vi "Teleop.vi"(9 "Teleop/Auto Cluster":T1={"x Joystick"={"Device"=enum."USB 0"}, "y Joystick"={"Device"=enum."USB 1"}, "controller"={"Device"=enum."USB 2"}, "right drive encoder"={"DevStatus"={"status"=FALSE, "code"=0, "source"=""}, "EncoderIndex"=enum."Enc 0", "CounterIndex"=enum."Invalid", "DistancePerCount"=1.0, "Decoding Type"=enum."4x"}, "left drive encoder"={"DevStatus"={"status"=FALSE, "code"=0, "source"=""}, "EncoderIndex"=enum."Enc 1", "CounterIndex"=enum."Invalid", "DistancePerCount"=1.0, "Decoding Type"=enum."4x"}, "drive motors"={"DevStatus"={"status"=FALSE, "code"=0, "source"=""}, "Motors[]"=[{"DeviceStatus"={"status"=FALSE, "code"=0, "source"=""}, "Type"=enum."CAN", "PWM"={"PWM Channel"=enum."Invalid", "DeadBand"={"Name"="", "maxPositivePwm"=0, "minPositivePwm"=0, "centerPwm"=0, "maxNegativePwm"=0, "minNegativePwm"=0, "angularRange"=0}}, "CAN"={"Device Number"=1, "SetOutput VI Ref"=variant(refnum<vi> refnum), "GetOutput VI Ref"=variant(refnum<vi> refnum), "Enable VI Ref"=variant(refnum<vi> refnum), "Disable VI Ref"=variant(refnum<vi> refnum), "Data"=variant(cluster{"Ext ID":u32, "Status 0 Session Handle":u32, "Status 1 Session Handle":u32, "Param Session Handle":u32, "Param Cache ref":refnum<data-value>, "CAN Timeout":u32, "Status 2 Session Handle":u32, "Status 3 Session Handle":u32, "Inverted No WPILib":bool, "Has Configured Limit Sw":bool, "Has Configured Alt Encoder":bool, "Status 4 Session Handle":u32} {"Ext ID"=33882113, "Status 0 Session Handle"=33965, "Status 1 Session Handle"=33966, "Param Session Handle"=33969, "Param Cache ref"=refnum, "CAN Timeout"=10, "Status 2 Session Handle"=33967, "Status 3 Session Handle"=33968, "Inverted No WPILib"=TRUE, "Has Configured Limit Sw"=FALSE, "Has Configured Alt Encoder"=FALSE, "Status 4 Session Handle"=0})}, "Invert"=FALSE, "DIO PWM"={"PWM \"Enable\" Channel"=enum."Invalid", "DIOChannel"=enum."Invalid", "PWM Rate"=0.0}}, {"DeviceStatus"={"status"=FALSE, "code"=0, "source"=""}, "Type"=enum."CAN", "PWM"={"PWM Channel"=enum."Invalid", "DeadBand"={"Name"="", "maxPositivePwm"=0, "minPositivePwm"=0, "centerPwm"=0, "maxNegativePwm"=0, "minNegativePwm"=0, "angularRange"=0}}, "CAN"={"Device Number"=3, "SetOutput VI Ref"=variant(refnum<vi> refnum), "GetOutput VI Ref"=variant(refnum<vi> refnum), "Enable VI Ref"=variant(refnum<vi> refnum), "Disable VI Ref"=variant(refnum<vi> refnum), "Data"=variant(cluster{"Ext ID":u32, "Status 0 Session Handle":u32, "Status 1 Session Handle":u32, "Param Session Handle":u32, "Param Cache ref":refnum<data-value>, "CAN Timeout":u32, "Status 2 Session Handle":u32, "Status 3 Session Handle":u32, "Inverted No WPILib":bool, "Has Configured Limit Sw":bool, "Has Configured Alt Encoder":bool, "Status 4 Session Handle":u32} {"Ext ID"=33882115, "Status 0 Session Handle"=33953, "Status 1 Session Handle"=33954, "Param Session Handle"=33957, "Param Cache ref"=refnum, "CAN Timeout"=10, "Status 2 Session Handle"=33955, "Status 3 Session Handle"=33956, "Inverted No WPILib"=FALSE, "Has Configured Limit Sw"=FALSE, "Has Configured Alt Encoder"=FALSE, "Status 4 Session Handle"=0})}, "Invert"=FALSE, "DIO PWM"={"PWM \"Enable\" Channel"=enum."Invalid", "DIOChannel"=enum."Invalid", "PWM Rate"=0.0}}], "Square Inputs"=FALSE, "Max Output"=1.0}, "gyro"={"DeviceStatus"={"status"=FALSE, "code"=0, "source"=""}, "Device Number"=0, "Type"=352321536, "Device ID"=352321536, "Handle"=3028580928, "UsageFrame"=0, "Library Path"=path "libCTRE_PhoenixCCI.so"}, "drive buttons"={"Device"=enum."USB 3"}} {"gyro"."Type" items=["CAN"=352321536, "TalonSRX"=33554432]}, 10 "Match Info":T16={"Autonomous Elapsed Seconds"=0.0, "TeleOp Elapsed Seconds"=13.899, "Disabled Elapsed Seconds"=41.877, "Visited Autonomous"=FALSE, "Visited TeleOp"=TRUE, "Visited Disabled"=TRUE, "Autonomous Settings"={"Autonomous Style"=enum."Independent", "VI Refnum"=refnum}}, 11 "Call Context":T17=enum."Stop") -> ()   [LabVIEW 2019]
doc: "This VI is called for each TeleOp packet received from the DS where the robot is not disabled. It is often used to read from the joysticks and update I/O or to update setpoints for timed control loops. It should complete and return within 20 milliseconds or it may miss DS packets."
uses:
  <vilib>/Rock Robotics/WPI/DriverStation/WPI_DriverStationDerivedRobotMode.ctl
  <vilib>/Rock Robotics/WPI/DriverStation/WPI_DriverStationMatch Info.ctl
  teleop auto cluster.ctl
  <vilib>/Rock Robotics/WPI/Joystick/WPI_JoystickDevRef.ctl
  <vilib>/Rock Robotics/WPI/Joystick/WPI_JoystickDeviceEnum.ctl
  <vilib>/Rock Robotics/WPI/Encoder/WPI_EncoderDevRef.ctl
  <vilib>/Rock Robotics/SystemInterfaces/Encoder/FPGA_EncoderIdx.ctl
  <vilib>/Rock Robotics/SystemInterfaces/Counter/FPGA_CounterCtrSystemIndex.ctl
  <vilib>/Rock Robotics/WPI/Encoder/WPI_EncoderType.ctl
  <vilib>/Rock Robotics/WPI/RobotDrive/WPI_RobotDriveDevRef.ctl
  <vilib>/Rock Robotics/WPI/MotorControl/WPI_MotorControlDeviceRef.ctl
  <vilib>/Rock Robotics/WPI/MotorControl/WPI_MotorControlType.ctl
  <vilib>/Rock Robotics/SystemInterfaces/DIO/FPGA_DIOPWMChannel.ctl
  <vilib>/Rock Robotics/WPI/PWM/WPI_PWMDeadband.ctl
  <vilib>/Rock Robotics/SystemInterfaces/DIO/FPGA_DIOChannel.ctl
  <vilib>/Rock Robotics/WPI/ThirdParty/Phoenix-LabVIEW/Pigeon IMU/CTRE_PigeonIMU_DeviceRef.ctl
  <vilib>/Rock Robotics/WPI/ThirdParty/Phoenix-LabVIEW/Pigeon IMU/CTRE_PigeonIMU_ConnectionType.ctl
  GlobalVariables.vi
  <vilib>/Rock Robotics/WPI/RobotDrive/WPI_RobotDriveArcadeDrive_Standard(NoSaturation).vi
panel:
  out "Static Setpoint":bool=TRUE
  in  "Elevator Manual":dbl=0.1
  # "false is layup\ntrue is trench shot"
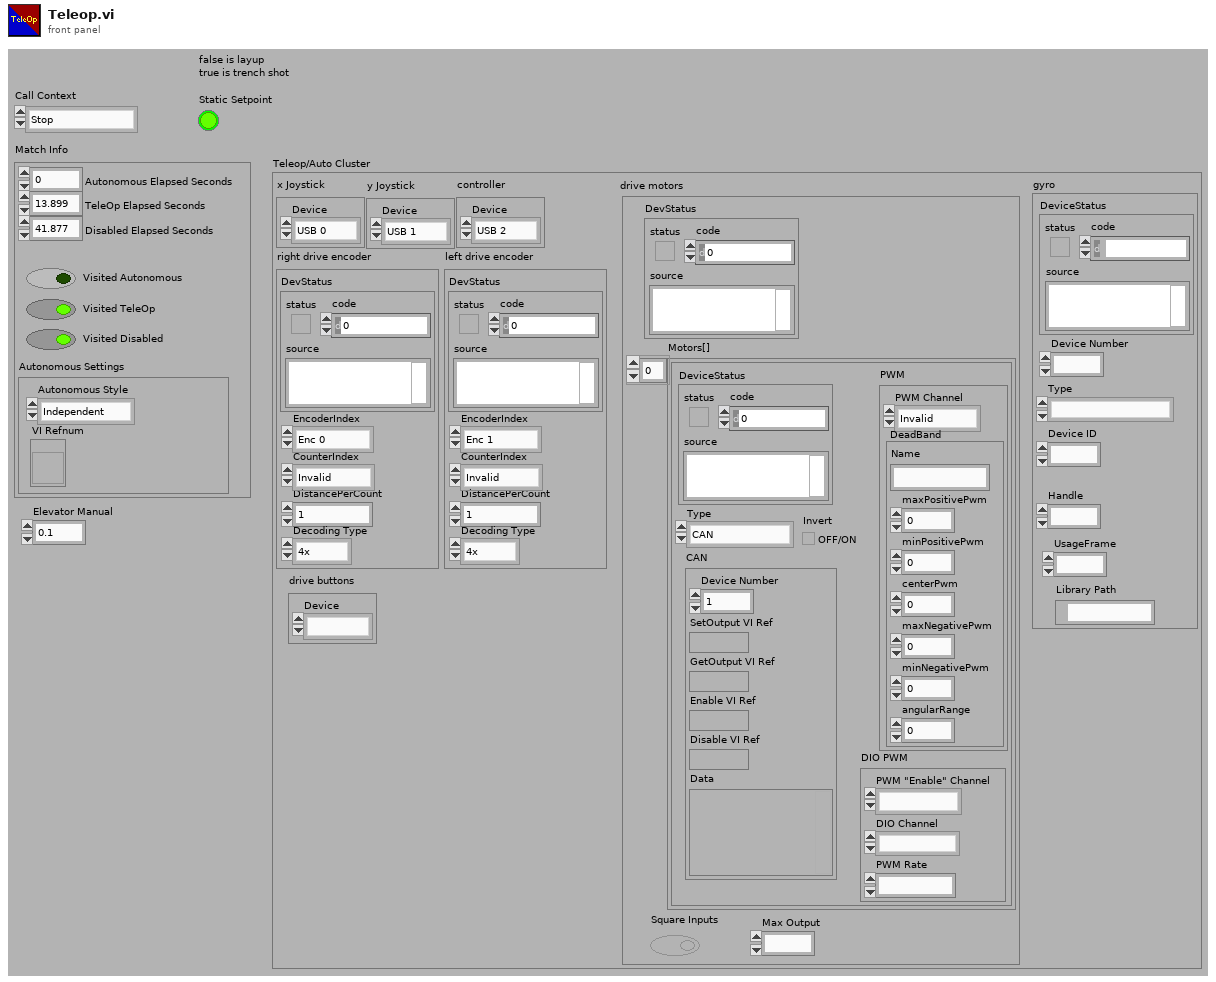
[diagram p1: front panel]
types:
  T1 = typedef "teleop auto cluster.ctl" = cluster{"x Joystick":T2, "y Joystick":T2, "controller":T2, "right drive encoder":T4, "left drive encoder":T4, "drive motors":T8, "gyro":T14, "drive buttons":T2}
  T2 = typedef "WPI_JoystickDevRef.ctl" = cluster{"Device":T3}
  T3 = typedef "WPI_JoystickDeviceEnum.ctl" = enum16{"USB 0", "USB 1", "USB 2", "USB 3", "USB 4", "USB 5"}
  T4 = typedef "WPI_EncoderDevRef.ctl" = cluster{"DevStatus":errorcluster, "EncoderIndex":T5, "CounterIndex":T6, "DistancePerCount":dbl, "Decoding Type":T7}
  T5 = typedef "FPGA_EncoderIdx.ctl" = enum8{"Enc 0", "Enc 1", "Enc 2", "Enc 3", "Enc 4", "Enc 5", "Enc 6", "Enc 7", "Invalid"}
  T6 = typedef "FPGA_CounterCtrSystemIndex.ctl" = enum8{"Ctr 0", "Ctr 1", "Ctr 2", "Ctr 3", "Ctr 4", "Ctr 5", "Ctr 6", "Ctr 7", "Invalid"}
  T7 = typedef "WPI_EncoderType.ctl" = enum16{"1x", "2x", "4x"}
  T8 = typedef "WPI_RobotDriveDevRef.ctl" = cluster{"DevStatus":errorcluster, "Motors[]":T9[], "Square Inputs":bool, "Max Output":dbl}
  T9 = typedef "WPI_MotorControlDeviceRef.ctl" = cluster{"DeviceStatus":errorcluster, "Type":T10, "PWM":cluster{"PWM Channel":T11, "DeadBand":T12}, "CAN":cluster{"Device Number":u8, "SetOutput VI Ref":variant, "GetOutput VI Ref":variant, "Enable VI Ref":variant, "Disable VI Ref":variant, "Data":variant}, "Invert":bool, "DIO PWM":cluster{"PWM \"Enable\" Channel":T11, "DIOChannel":T13, "PWM Rate":dbl}}
  T10 = typedef "WPI_MotorControlType.ctl" = enum16{"PWM", "CAN", "DIO PWM"}
  T11 = typedef "FPGA_DIOPWMChannel.ctl" = enum8{"PWM 0", "PWM 1", "PWM 2", "PWM 3", "PWM 4", "PWM 5", "PWM 6", "PWM 7", "PWM 8", "PWM 9", "PWM MXP 0", "PWM MXP 1", "PWM MXP 2", "PWM MXP 3", "PWM MXP 4", "PWM MXP 5", "PWM MXP 6", "PWM MXP 7", "PWM MXP 8", "PWM MXP 9", "Invalid"}
  T12 = typedef "WPI_PWMDeadband.ctl" = cluster{"Name":string, "maxPositivePwm":i32, "minPositivePwm":i32, "centerPwm":i32, "maxNegativePwm":i32, "minNegativePwm":i32, "angularRange":u16}
  T13 = typedef "FPGA_DIOChannel.ctl" = enum8{"DIO 0", "DIO 1", "DIO 2", "DIO 3", "DIO 4", "DIO 5", "DIO 6", "DIO 7", "DIO 8", "DIO 9", "DIO MXP 0", "DIO MXP 1", "DIO MXP 2", "DIO MXP 3", "DIO MXP 4", "DIO MXP 5", "DIO MXP 6", "DIO MXP 7", "DIO MXP 8", "DIO MXP 9", "DIO MXP 10", "DIO MXP 11", "DIO MXP 12", "DIO MXP 13", "DIO MXP 14", "DIO MXP 15", "SPI Port CS1", "SPI Port CS2", "SPI Port CS3", "SPI Port MISO", "SPI Port MOSI", "Invalid"}
  T14 = typedef "CTRE_PigeonIMU_DeviceRef.ctl" = cluster{"DeviceStatus":errorcluster, "Device Number":u8, "Type":T15, "Device ID":u32, "Handle":u64, "UsageFrame":u32, "Library Path":path}
  T15 = typedef "CTRE_PigeonIMU_ConnectionType.ctl" = u32
  T16 = typedef "WPI_DriverStationMatch Info.ctl" = cluster{"Autonomous Elapsed Seconds":dbl, "TeleOp Elapsed Seconds":dbl, "Disabled Elapsed Seconds":dbl, "Visited Autonomous":bool, "Visited TeleOp":bool, "Visited Disabled":bool, "Autonomous Settings":cluster{"Autonomous Style":enum16{"Iterative", "Independent"}, "VI Refnum":refnum<vi>}}
  T17 = typedef "WPI_DriverStationDerivedRobotMode.ctl" = enum16{"Init", "Execute", "Stop"}
  T18 = enum16{"ground protect", "ground pickup", "control panel", "shooting", "climb", "unjam", "intake shoot"}
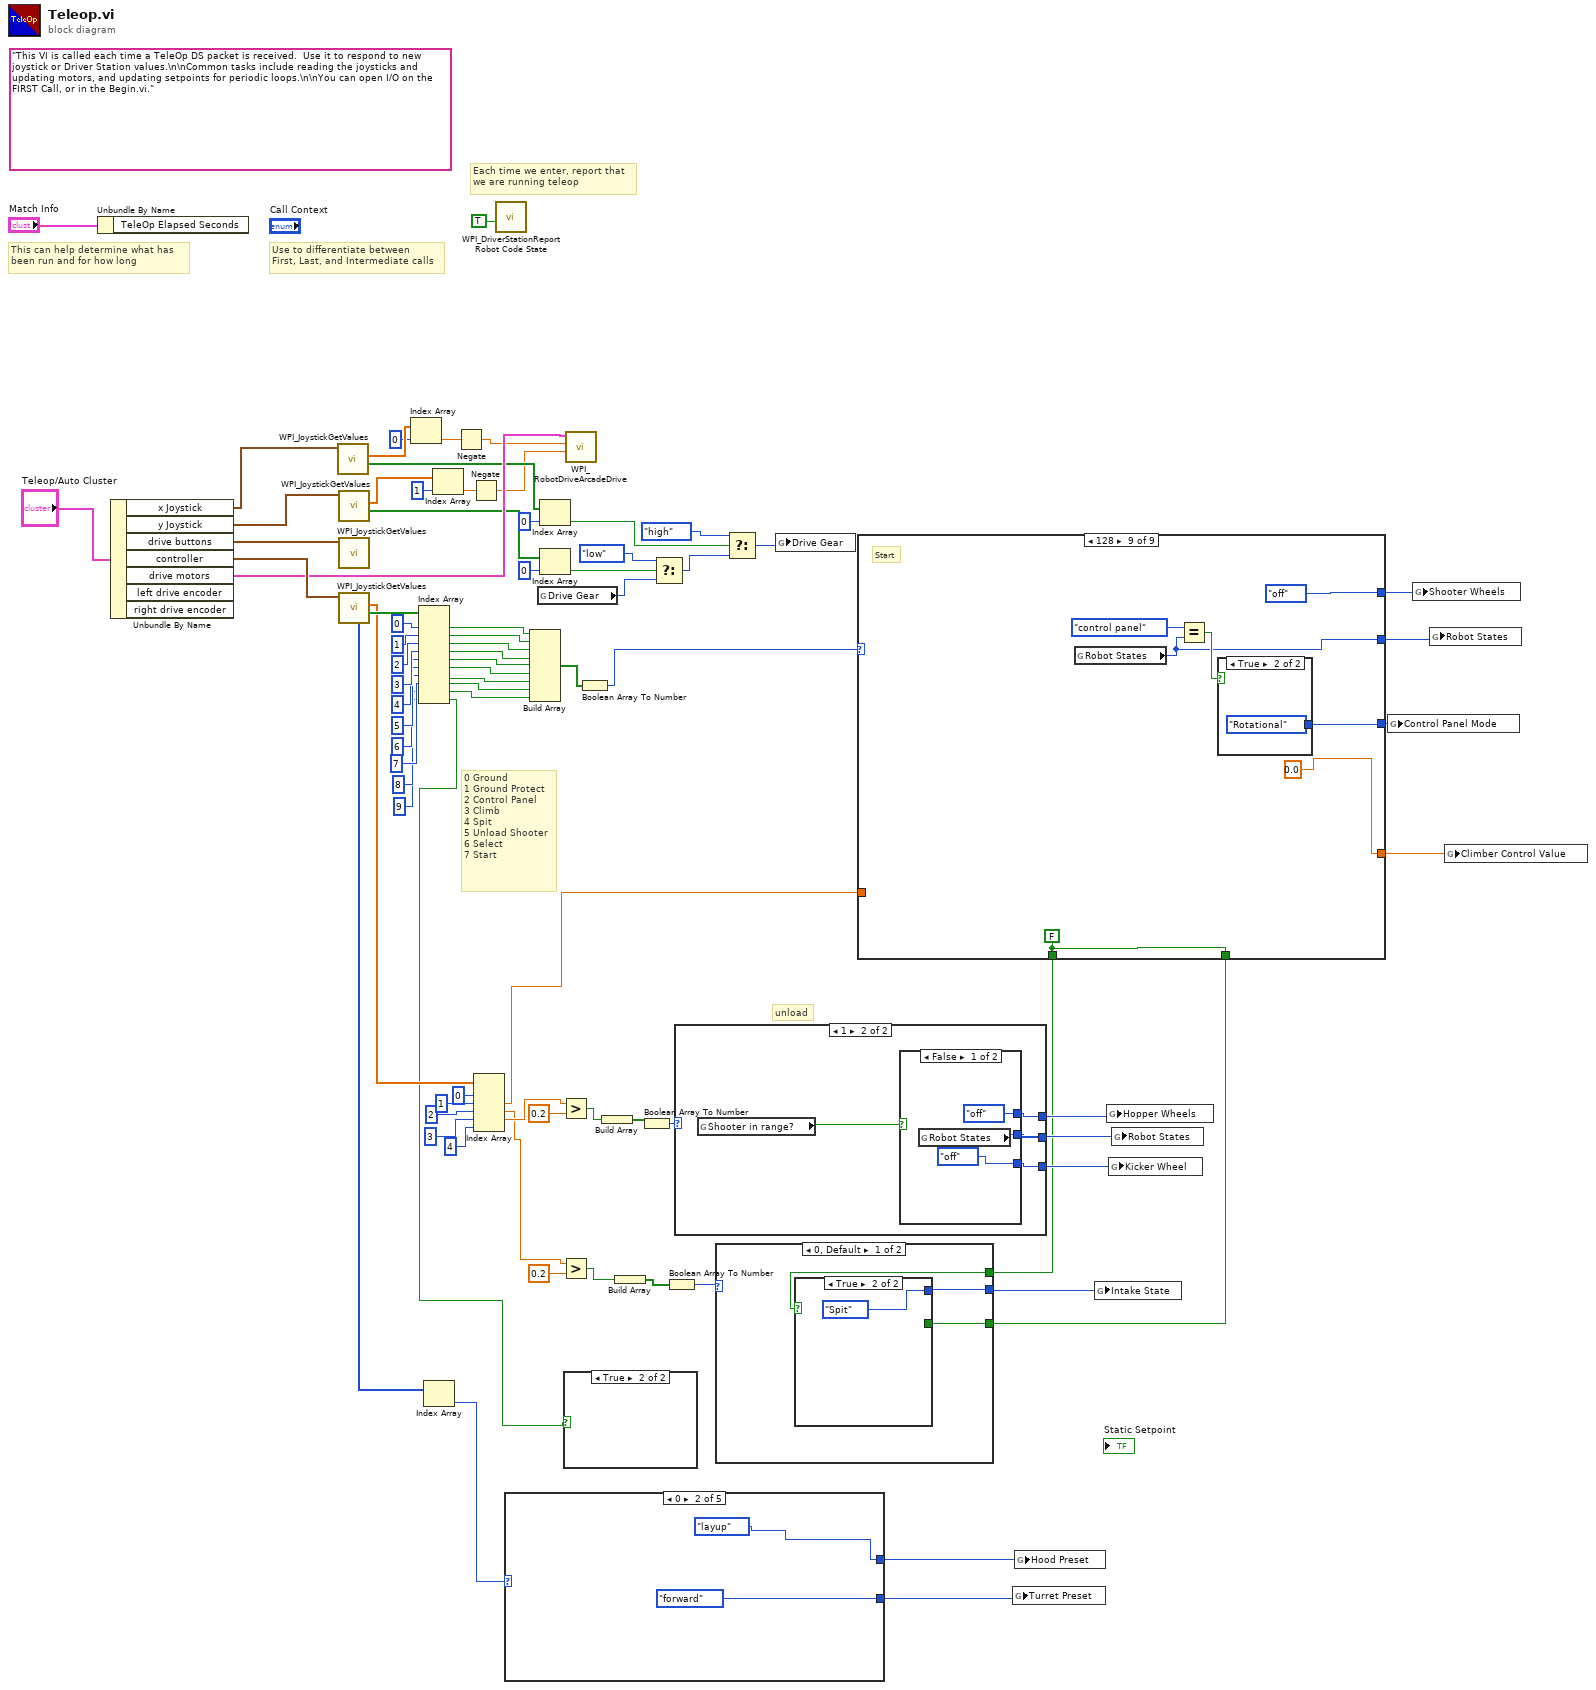
[diagram p0: block diagram]
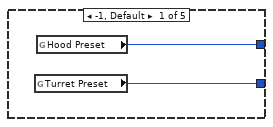
[diagram p3: hidden frame]
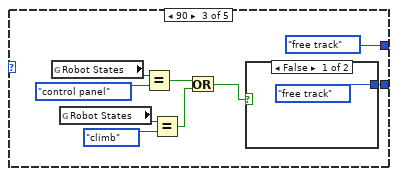
[diagram p4: hidden frame]
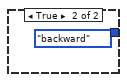
[diagram p5: hidden frame]
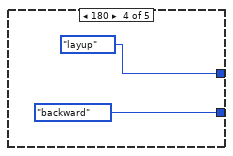
[diagram p6: hidden frame]
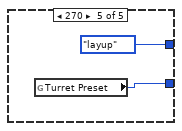
[diagram p7: hidden frame]
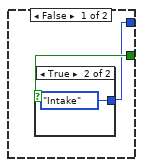
[diagram p8: hidden frame]
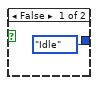
[diagram p9: hidden frame]
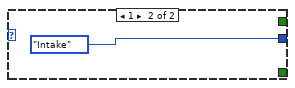
[diagram p10: hidden frame]
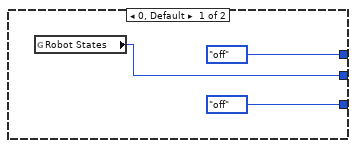
[diagram p11: hidden frame]
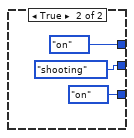
[diagram p12: hidden frame]
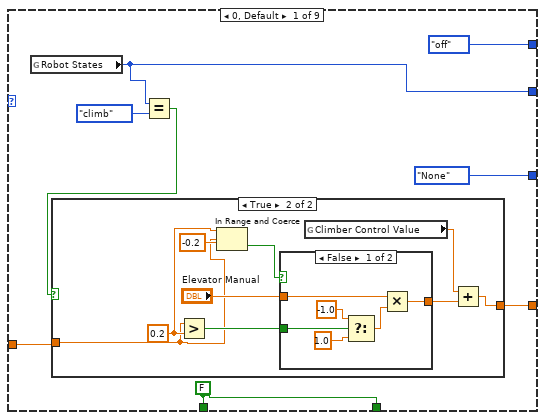
[diagram p13: hidden frame]
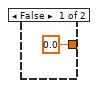
[diagram p14: hidden frame]
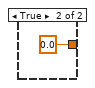
[diagram p15: hidden frame]
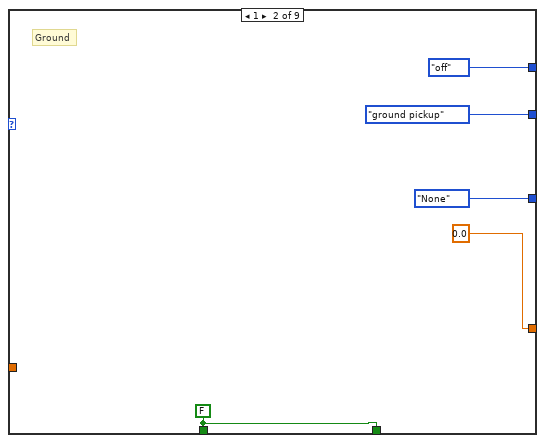
[diagram p16: hidden frame]
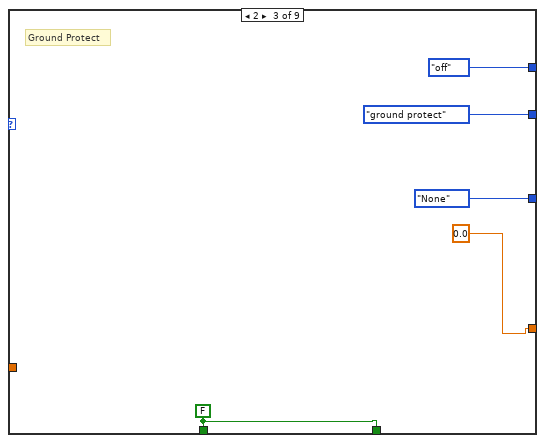
[diagram p17: hidden frame]
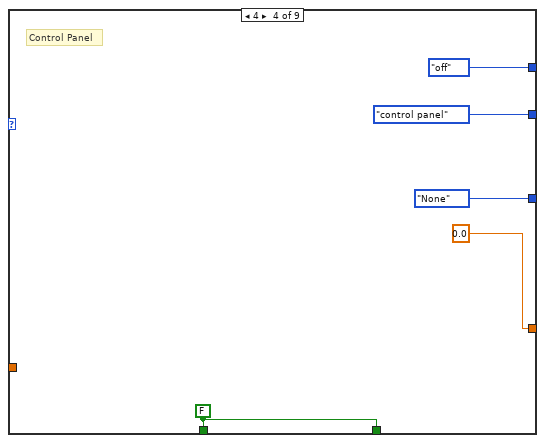
[diagram p18: hidden frame]
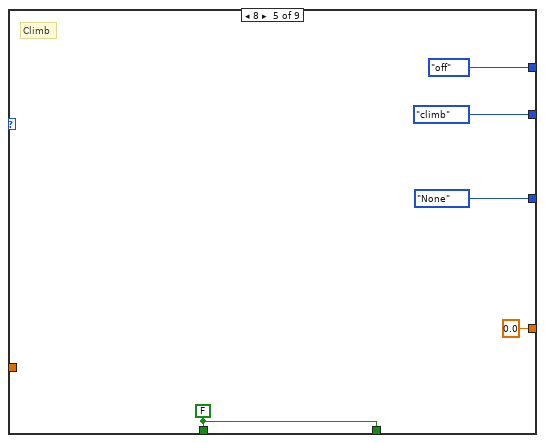
[diagram p19: hidden frame]
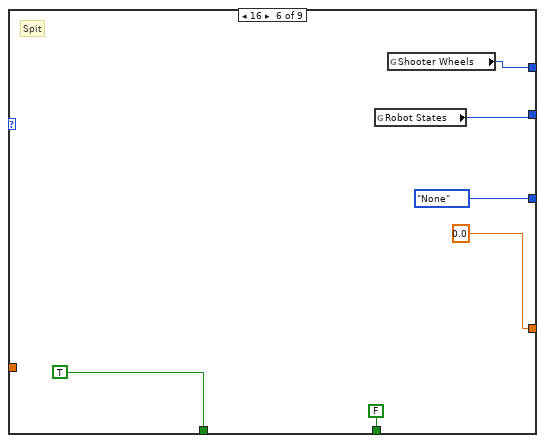
[diagram p20: hidden frame]
diagram:
  (unwired) "This VI is called each time a TeleOp DS packet is received.  Use it to respond to new joystick or Driver Station values.\n\nCommon tasks include reading the joysticks and updating motors, and updating setpoints for periodic loops.\n\nYou can open I/O on the FIRST Call, or in the Begin.vi."
  # "unload"
  # "0 Ground\n1 Ground Protect\n2 Control Panel\n3 Climb\n4 Spit\n5 Unload Shooter\n6 Select\n7 Start"
  # "Each time we enter, report that\nwe are running teleop"
  # "Use to differentiate between\nFirst, Last, and Intermediate calls"
  # "This can help determine what has\nbeen run and for how long"
  n1 = Unbundle By Name("Match Info") -> ()  [unwired: 1 out]
  n2 = Unbundle By Name("Teleop/Auto Cluster") -> ("x Joystick"=w78:T2, "y Joystick"=w77:T2, "drive buttons"=w76:T2, "controller"=w75:T2, "drive motors"=w70:T8)  [unwired: 2 out]
  n3 = call <vilib>:"WPI_JoystickGetValues.vi"("JoystickDevRef"=w78) -> ("Buttons"=w69:bool[], "Axes"=w72:dbl[])  [unwired: 6 in, 3 out]
  n4 = call <vilib>:"WPI_JoystickGetValues.vi"("JoystickDevRef"=w77) -> ("Buttons"=w68:bool[], "Axes"=w74:dbl[])  [unwired: 6 in, 3 out]
  n5 = call <vilib>:"WPI_JoystickGetValues.vi"("JoystickDevRef"=w76) -> ()  [unwired: 6 in, 5 out]
  n6 = call <vilib>:"WPI_JoystickGetValues.vi"("JoystickDevRef"=w75) -> ("Buttons"=w58:bool[], "Axes"=w37:dbl[], "POVs"=w31:i16[])  [unwired: 6 in, 2 out]
  n7 = Index Array(array=w72, index=0) -> (element=w17:dbl)
  n8 = Index Array(array=w58, index #1=0 ("index"), index #2=1 ("index"), index #3=2 ("index"), index #4=3 ("index"), index #5=4 ("index"), index #6=5 ("index"), index #7=6 ("index"), index #8=7 ("index"), index #9=8 ("index"), index #10=9 ("index")) -> (element #1=w49:bool, element #2=w48:bool, element #3=w45:bool, element #4=w44:bool, element #5=w43:bool, element #6=w41:bool, element #7=w40:bool, element #8=w39:bool, element #9=w38:bool, element #10=w1:bool)
  n9 = Index Array(array=w31) -> (element=w13:i16)  [unwired: 1 in]
  n10 = Index Array(array=w74, index=1) -> (element=w18:dbl)
  n11 = Negate(x=w17) -> (-x=w14:dbl)
  n12 = Negate(x=w18) -> (-x=w16:dbl)
  n13 = Index Array(array=w37, index #1=0 ("index"), index #2=1 ("index"), index #3=2 ("index"), index #4=3 ("index"), index #5=4 ("index")) -> (element #2=w5:dbl, element #3=w15:dbl, element #4=w22:dbl)  [unwired: 2 out]
  n14 = call <vilib>:"WPI_DriverStationReport Robot Code State.vi"("TeleOp"=TRUE ("Autonomous")) -> ()  [unwired: 10 in, 1 out]
  n15 = case shown="0" w13 {
    tunnel: [w83 enum16{"free track", "forward", "backward"}."forward" ("Turret Preset") w94 enum16{"free track", "forward", "backward"}."backward" ("Turret Preset") w99] -> w12
    tunnel: [w82 enum16{"trench", "layup", "free track"}."layup" ("Hood Preset") enum16{"trench", "layup", "free track"}."free track" ("Hood Preset") enum16{"trench", "layup", "free track"}."layup" ("Hood Preset") enum16{"trench", "layup", "free track"}."layup" ("Hood Preset")] -> w11
    frame -1, Default {
      n16 = global read "GlobalVariables.vi" "Turret Preset"() -> (w83:enum16{"free track", "forward", "backward"})
      n17 = global read "GlobalVariables.vi" "Hood Preset"() -> (w82:enum16{"trench", "layup", "free track"})
    }
    frame 0 {
    }
    frame 90 {
      n18 = global read "GlobalVariables.vi" "Robot States"() -> (w92:T18)
      n19 = global read "GlobalVariables.vi" "Robot States"() -> (w88:T18)
      n20 = Equal?(x=w92, y=T18."control panel") -> (x = y?=w90:bool)
      n21 = Equal?(x=w88, y=T18."climb") -> (x = y?=w87:bool)
      n22 = Or(x=w90, y=w87) -> (x .or. y?=w86:bool)
      n23 = case shown="False" w86 {
        tunnel: [enum16{"free track", "forward", "backward"}."free track" ("Turret Preset") enum16{"free track", "forward", "backward"}."backward" ("Turret Preset")] -> w94
        frame False {
        }
        frame True {
        }
      }
    }
    frame 180 {
    }
    frame 270 {
      n24 = global read "GlobalVariables.vi" "Turret Preset"() -> (w99:enum16{"free track", "forward", "backward"})
    }
  }
  n25 = Build Array(w49, w48, w45, w44, w43, w41, w40, w39, w38) -> (w47:bool[])
  n26 = global read "GlobalVariables.vi" "Drive Gear"() -> (w64:enum16{"high", "low"})
  n27 = Index Array(array=w69, index=0) -> (element=w61:bool)
  n28 = Index Array(array=w68, index=0) -> (element=w65:bool)
  n29 = Greater?(x=w22, y=0.2) -> (0:w7:bool)
  n30 = Greater?(x=w15, y=0.2) -> (0:w6:bool)
  n31 = case shown="True" w1 {
    frame False {
    }
    frame True {
    }
  }
  n32 = call-poly <vilib>:"WPI_RobotDriveArcadeDrive.vi"("Y axis value"=w16, "X axis value"=w14, "RobotDriveDevRef"=w70) -> ()  [unwired: 6 in, 3 out]
  n33 = Boolean Array To Number(Boolean array=w47) -> (number=w46:u32)
  n34 = Build Array(w7) -> (w35:bool[])
  n35 = Build Array(w6) -> (w30:bool[])
  n36 = Boolean Array To Number(Boolean array=w35) -> (number=w34:u32)
  n37 = Select(t=enum16{"high", "low"}."low", s=w65, f=w64) -> (s? t:f=w62:enum16{"high", "low"})
  n38 = Boolean Array To Number(Boolean array=w30) -> (number=w28:u32)
  n39 = case shown="1" w34 {
    tunnel: [w103 w104] -> w33
    tunnel: [enum16{"on", "off"}."off" ("Hopper Wheels") w106] -> w9
    tunnel: [enum16{"on", "off", "reverse"}."off" ("Kicker Wheel") w105] -> w8
    frame 0, Default {
      n40 = global read "GlobalVariables.vi" "Robot States"() -> (w103:T18)
    }
    frame 1 {
      n41 = global read "GlobalVariables.vi" "Shooter in range?"() -> (w107:bool)
      n42 = case shown="False" w107 {
        tunnel: [enum16{"on", "off"}."off" ("Hopper Wheels") enum16{"on", "off"}."on" ("Hopper Wheels")] -> w106
        tunnel: [enum16{"on", "off", "reverse"}."off" ("Kicker Wheel") enum16{"on", "off", "reverse"}."on" ("Kicker Wheel")] -> w105
        tunnel: [w108 T18."shooting" ("Robot States")] -> w104
        frame False {
          n43 = global read "GlobalVariables.vi" "Robot States"() -> (w108:T18)
        }
        frame True {
        }
      }
    }
  }
  n44 = Select(t=enum16{"high", "low"}."high", s=w61, f=w62) -> (s? t:f=w59:enum16{"high", "low"})
  n45 = global write "GlobalVariables.vi" "Drive Gear"(w59) -> ()
  n46 = case shown="128" w46 {
    tunnel: [w117 T18."ground pickup" ("Robot States") T18."ground protect" ("Robot States") T18."control panel" ("Robot States") T18."climb" ("Robot States") w162 w168 w173 w183] -> w42
    tunnel: [enum16{"on", "off"}."off" ("Shooter Wheels") enum16{"on", "off"}."off" ("Shooter Wheels") enum16{"on", "off"}."off" ("Shooter Wheels") enum16{"on", "off"}."off" ("Shooter Wheels") enum16{"on", "off"}."off" ("Shooter Wheels") w161 enum16{"on", "off"}."on" ("Shooter Wheels") enum16{"on", "off"}."off" ("Shooter Wheels") enum16{"on", "off"}."off" ("Shooter Wheels")] -> w32
    tunnel: [enum16{"Rotational", "None", "Posistional"}."None" ("Control Panel Mode") enum16{"Rotational", "None", "Posistional"}."None" ("Control Panel Mode") enum16{"Rotational", "None", "Posistional"}."None" ("Control Panel Mode") enum16{"Rotational", "None", "Posistional"}."None" ("Control Panel Mode") enum16{"Rotational", "None", "Posistional"}."None" ("Control Panel Mode") enum16{"Rotational", "None", "Posistional"}."None" ("Control Panel Mode") enum16{"Rotational", "None", "Posistional"}."None" ("Control Panel Mode") w175 w181] -> w10
    tunnel: w5 -> [w119 _ _ _ _ _ _ _ _]
    tunnel: [w118 0.0 0.0 0.0 0.0 0.0 0.0 0.0 0.0] -> w4
    tunnel: [w114 w139 w144 w149 w154 TRUE w165 FALSE w179] -> w3
    tunnel: [w114 w139 w144 w149 w154 FALSE w165 w170 w179] -> w2
    frame 0, Default {
      w114 = FALSE
      n47 = global read "GlobalVariables.vi" "Robot States"() -> (w117:T18)
      n48 = Equal?(x=w117, y=T18."climb") -> (x = y?=w115:bool)
      n49 = case shown="True" w115 {
        tunnel: w119 -> [_ w124]
        tunnel: [0.0 w123] -> w118
        frame False {
        }
        frame True {
          w126 = 0.2 ("y")
          n50 = Greater?(x=w124, y=w126) -> (0:w128:bool)
          n51 = In Range and Coerce(upper limit=w126, x=w124, lower limit=-0.2 ("y")) -> (In Range?=w129:bool)  [unwired: 1 out]
          n52 = case shown="False" w129 {
            tunnel: [w134 0.0] -> w127
            tunnel: "Elevator Manual" -> [w137 _]
            tunnel: w128 -> [w132 _]
            frame False {
              n53 = Select(t=-1.0, s=w132, f=1.0) -> (s? t:f=w133:dbl)
              n54 = Multiply(x=w137, y=w133) -> (x*y=w134:dbl)
            }
            frame True {
            }
          }
          n55 = global read "GlobalVariables.vi" "Climber Control Value"() -> (w131:dbl)
          n56 = Add(x=w131, y=w127) -> (x+y=w123:dbl)
        }
      }
    }
    frame 1 {
      w139 = FALSE
      # "Ground"
    }
    frame 2 {
      w144 = FALSE
      # "Ground Protect"
    }
    frame 4 {
      w149 = FALSE
      # "Control Panel"
    }
    frame 8 {
      w154 = FALSE
      # "Climb"
    }
    frame 16 {
      # "Spit"
      n57 = global read "GlobalVariables.vi" "Robot States"() -> (w162:T18)
      n58 = global read "GlobalVariables.vi" "Shooter Wheels"() -> (w161:enum16{"on", "off"})
    }
    frame 32 {
      w165 = FALSE
      # "Unload Shooter"
      n59 = global read "GlobalVariables.vi" "Robot States"() -> (w168:T18)
    }
    frame 64 {
      # "Select"
      n60 = global read "GlobalVariables.vi" "Robot States"() -> (w173:T18)
      n61 = Equal?(x=T18."control panel", y=w173) -> (x = y?=w170:bool)
      n62 = case shown="True" w170 {
        tunnel: [enum16{"Rotational", "None", "Posistional"}."None" ("Control Panel Mode") enum16{"Rotational", "None", "Posistional"}."Posistional" ("Control Panel Mode")] -> w175
        frame False {
        }
        frame True {
        }
      }
    }
    frame 128 {
      w179 = FALSE
      # "Start"
      n63 = global read "GlobalVariables.vi" "Robot States"() -> (w183:T18)
      n64 = Equal?(x=T18."control panel", y=w183) -> (x = y?=w184:bool)
      n65 = case shown="True" w184 {
        tunnel: [enum16{"Rotational", "None", "Posistional"}."None" ("Control Panel Mode") enum16{"Rotational", "None", "Posistional"}."Rotational" ("Control Panel Mode")] -> w181
        frame False {
        }
        frame True {
        }
      }
    }
  }
  n66 = case shown="0, Default" w28 {
    tunnel: [w190 enum16{"Idle", "Intake", "Spit"}."Intake" ("Intake State")] -> w21
    tunnel: w3 -> [w189 _]
    tunnel: w2 -> [w188 _]
    frame 0, Default {
      n67 = case shown="True" w189 {
        tunnel: [w191 enum16{"Idle", "Intake", "Spit"}."Spit" ("Intake State")] -> w190
        tunnel: w188 -> [w192 _]
        frame False {
          n68 = case shown="True" w192 {
            tunnel: [enum16{"Idle", "Intake", "Spit"}."Idle" ("Intake State") enum16{"Idle", "Intake", "Spit"}."Intake" ("Intake State")] -> w191
            frame False {
            }
            frame True {
            }
          }
        }
        frame True {
        }
      }
    }
    frame 1 {
    }
  }
  n69 = global write "GlobalVariables.vi" "Turret Preset"(w12) -> ()
  n70 = global write "GlobalVariables.vi" "Hood Preset"(w11) -> ()
  n71 = global write "GlobalVariables.vi" "Intake State"(w21) -> ()
  n72 = global write "GlobalVariables.vi" "Hopper Wheels"(w9) -> ()
  n73 = global write "GlobalVariables.vi" "Kicker Wheel"(w8) -> ()
  n74 = global write "GlobalVariables.vi" "Robot States"(w33) -> ()
  n75 = global write "GlobalVariables.vi" "Control Panel Mode"(w10) -> ()
  n76 = global write "GlobalVariables.vi" "Shooter Wheels"(w32) -> ()
  n77 = global write "GlobalVariables.vi" "Robot States"(w42) -> ()
  n78 = global write "GlobalVariables.vi" "Climber Control Value"(w4) -> ()
